vi "Check router handshake for errors.vi"(8 "error in":errorcluster, 11 "Bytes (in)":u8[](array[numeric])) -> (0 "error out":errorcluster, 3 "Byte (out)":u8[](array[numeric]))   [LabVIEW 2020, in "wamplv.lvlib" / "RawSocket TCP Handler.lvclass"]
uses:
  RawSocket TCP Handler.lvclass
  RawSocket TCP Handler.lvclass/RawSocket TCP Handler.ctl
  <vilib>/Utility/error.llb/Error Cluster From Error Code.vi
  <vilib>/ErrorRing/Error Ring.xnode
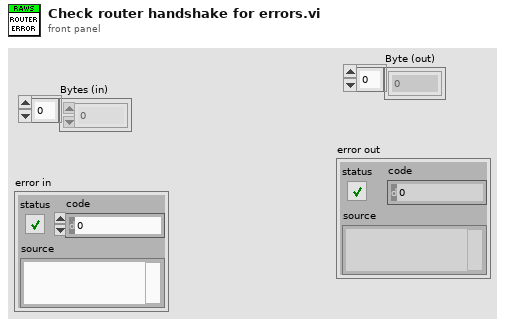
[diagram p1: front panel]
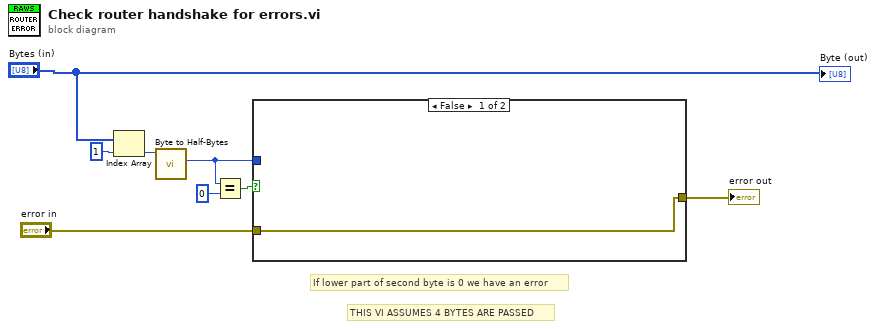
[diagram p0: block diagram]
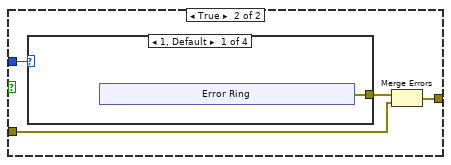
[diagram p2: hidden frame]
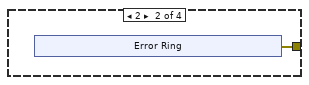
[diagram p3: hidden frame]
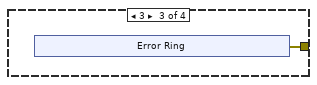
[diagram p4: hidden frame]
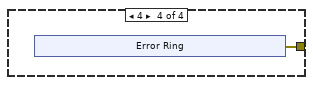
[diagram p5: hidden frame]
diagram:
  # "If lower part of second byte is 0 we have an error"
  # "THIS VI ASSUMES 4 BYTES ARE PASSED"
  n1 = Index Array(array="Bytes (in)", index=1) -> (element=w4:u8)
  n2 = call "Byte to Half-Bytes.vi"("Byte In"=w4) -> ("Lower Half-byte"=w1:u8)  [unwired: 7 in, 1 out]
  n3 = Equal?(x=w1, y=u8 0) -> (x = y?=w2:bool)
  n4 = case shown="False" w2 {
    tunnel: w1 -> [_ w11]
    tunnel: "error in" -> [w9 w12]
    tunnel: [w9 w13] -> w6
    frame False {
    }
    frame True {
      n5 = case shown="1, Default" w11 {
        tunnel: [w14 w19 w24 w29] -> w10
        frame 1, Default {
          n6 = xnode "Error Ring"() -> ("error out"=w14:errorcluster)
        }
        frame 2 {
          n7 = xnode "Error Ring"() -> ("error out"=w19:errorcluster)
        }
        frame 3 {
          n8 = xnode "Error Ring"() -> ("error out"=w24:errorcluster)
        }
        frame 4 {
          n9 = xnode "Error Ring"() -> ("error out"=w29:errorcluster)
        }
      }
      n10 = Merge Errors(w10, w12) -> (w13:errorcluster)
    }
  }
  "error out" <- w6
  "Byte (out)" <- "Bytes (in)"
